vi "Query Sequencer ARB File All Sample Rates.vi"(8 "error in (no error)":errorcluster, 10 "Instance (1)":i32=1, 11 "VISA resource name":refnum<visa-resource-name>) -> (0 "error out":errorcluster, 2 "Sample Rates":i32[](array[numeric]), 3 "VISA resource name out":refnum<visa-resource-name>)   [LabVIEW 2020, in "Rohde&Schwarz CMXP GPRF.lvlib"]
doc: "Queries the sample rates of all ARB files.\n\nAttribute:\nRSCMXPGPRF_ATTR_SEQUENCER_ARB_FILE_ALL_SAMPLE_RATES\n\nRemote-control command:\nSOURce:GPRF:GEN<i>:SEQuencer:APOol:SRATe:ALL?"
uses:
  <instrlib>/Rohde&Schwarz CMXP GPRF/Rohde&Schwarz CMXP GPRF.lvlib
  <instrlib>/Rohde&Schwarz CMXP GPRF/Private/rsidr_core.llb/rsidr_core.lvlib
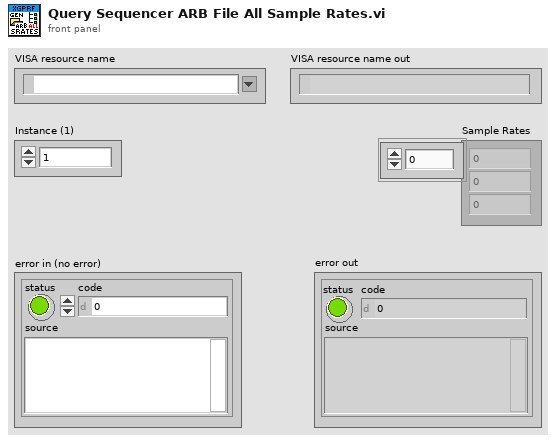
[diagram p1: front panel]
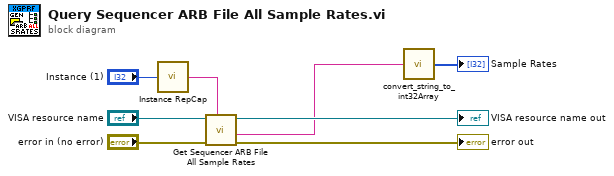
[diagram p0: block diagram]
diagram:
  n1 = call <instrlib>:"Instance RepCap.vi"("Instance in"="Instance (1)") -> ("Instance out"=w2:string)
  n2 = call "Get Sequencer ARB File All Sample Rates"("Repeated Capabilities"=w2, "error in (no error)"="error in (no error)", "instrument handle"="VISA resource name") -> ("error out"=→"error out":errorcluster, "Sequencer ARB File All Sample Rates"=w1:string, "instrument handle out"=→"VISA resource name out":refnum<visa-resource-name>)  [unwired: 6 in]
  n3 = call <instrlib>:"convert_string_to_int32Array.vi"("string in"=w1) -> ("int32 array out"=→"Sample Rates":i32[])  [unwired: 3 in, 1 out]
